vi "Get IO Nodes.vi"(8 "error in (no error)":errorcluster, 11 "DAQ in":refnum<class "DAQ.lvclass">) -> (0 "error out":errorcluster, 2 "IO Nodes":T1 {"AO Config"."AO Channels"."Conversion"."ScaleOffset" format="%.3f"; "AO Config"."AO Channels"."Conversion"."MinEngUnit" format="%.3f"; "AO Config"."AO Channels"."Conversion"."MaxEngUnit" format="%.3f"; "AO Config"."AO Channels"."Conversion"."MinSignal" format="%.3f"; "AO Config"."AO Channels"."Conversion"."MaxSignal" format="%.3f"; "AI Config"."AI Tasks"."AI Channels"."Conversion"."ScaleOffset" format="%.3f"; "AI Config"."AI Tasks"."AI Channels"."Conversion"."MinEngUnit" format="%.3f"; "AI Config"."AI Tasks"."AI Channels"."Conversion"."MaxEngUnit" format="%.3f"; "AI Config"."AI Tasks"."AI Channels"."Conversion"."MinSignal" format="%.3f"; "AI Config"."AI Tasks"."AI Channels"."Conversion"."MaxSignal" format="%.3f"; "AI Config"."AI Tasks"."AI Channels"."Terminal Configuration" items=["default"=-1, "RSE"=10083, "NRSE"=10078, "Differential"=10106, "Pseudodifferential"=12529]}, 3 "DAQ out":refnum<class "DAQ.lvclass">)   [LabVIEW 2017, in "DAQ.lvclass"]
doc: "Developed by Kevin Thompson\nkevin@thompsonengineering.net\n\nCopyright 2018-2020\nThompson Engineering, LLC"
uses:
  DAQ.lvclass
  DataTypes/TD IO Node Definition--cluster.ctl
  DataTypes/TD DI Config--cluster.ctl
  DataTypes/TD DI Task--cluster.ctl
  DataTypes/TD DI Channel--cluster.ctl
  DataTypes/TD DO Config--cluster.ctl
  DataTypes/TD DO Channel--cluster.ctl
  DataTypes/TD AI Config--cluster.ctl
  DataTypes/TD AI Task--cluster.ctl
  DataTypes/TD AI Channel--cluster.ctl
  DataTypes/TD DataValueConversion--cluster.ctl
  DataTypes/TD AI DAQ Type--enum.ctl
  DataTypes/TD AI Force Bridge--cluster.ctl
  DataTypes/TD AO Config--cluster.ctl
  DataTypes/TD AO Channel--cluster.ctl
  DAQ.lvclass/DAQ.ctl
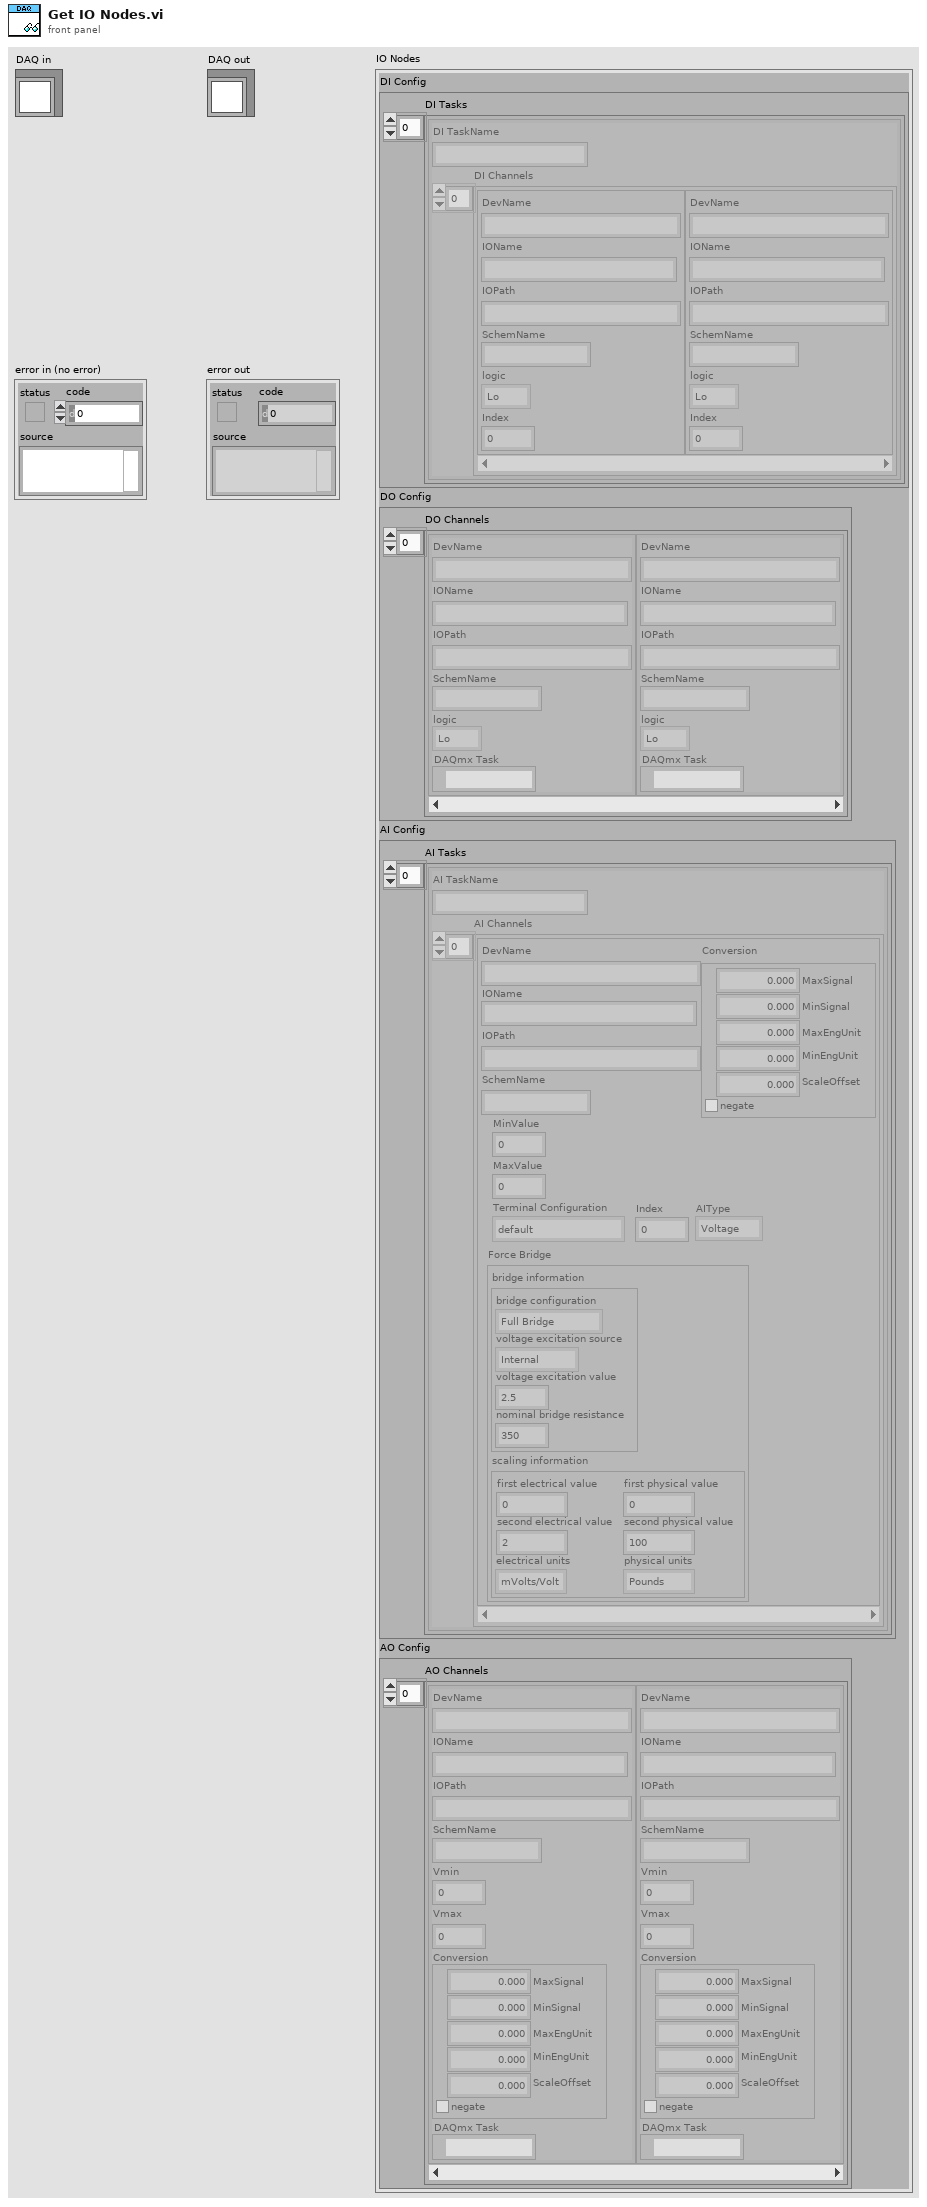
[diagram p1: front panel]
types:
  T1 = typedef "DAQ.lvclass/TD IO Node Definition--cluster.ctl" = cluster{"DI Config":T2, "DO Config":T5, "AI Config":T7, "AO Config":T13}
  T2 = typedef "DAQ.lvclass/TD DI Config--cluster.ctl" = cluster{"DI Tasks":T3[]}
  T3 = typedef "DAQ.lvclass/TD DI Task--cluster.ctl" = cluster{"DI TaskName":string, "DI Channels":T4[]}
  T4 = typedef "DAQ.lvclass/TD DI Channel--cluster.ctl" = cluster{"DevName":string, "IOName":string, "IOPath":string, "SchemName":string, "logic":enum16{"Lo", "Hi"}, "Index":i32}
  T5 = typedef "DAQ.lvclass/TD DO Config--cluster.ctl" = cluster{"DO Channels":T6[]}
  T6 = typedef "DAQ.lvclass/TD DO Channel--cluster.ctl" = cluster{"DevName":string, "IOName":string, "IOPath":string, "SchemName":string, "logic":enum16{"Lo", "Hi"}, "DAQmx Task":refnum<k21>}
  T7 = typedef "DAQ.lvclass/TD AI Config--cluster.ctl" = cluster{"AI Tasks":T8[]}
  T8 = typedef "DAQ.lvclass/TD AI Task--cluster.ctl" = cluster{"AI TaskName":string, "AI Channels":T9[]}
  T9 = typedef "DAQ.lvclass/TD AI Channel--cluster.ctl" = cluster{"DevName":string, "IOName":string, "IOPath":string, "SchemName":string, "MinValue":dbl, "MaxValue":dbl, "Terminal Configuration":i32, "Index":i32, "Conversion":T10, "AIType":T11, "Force Bridge":T12}
  T10 = typedef "DAQ.lvclass/TD DataValueConversion--cluster.ctl" = cluster{"MaxSignal":dbl, "MinSignal":dbl, "MaxEngUnit":dbl, "MinEngUnit":dbl, "ScaleOffset":dbl, "negate":bool}
  T11 = typedef "DAQ.lvclass/TD AI DAQ Type--enum.ctl" = enum16{"Voltage", "Current", "Strain Gage", "Force Bridge"}
  T12 = typedef "DAQ.lvclass/TD AI Force Bridge--cluster.ctl" = cluster{"bridge information":cluster{"bridge configuration":i32, "voltage excitation source":i32, "voltage excitation value":dbl, "nominal bridge resistance":dbl}, "scaling information":cluster{"first electrical value":dbl, "second electrical value":dbl, "electrical units":i32, "first physical value":dbl, "second physical value":dbl, "physical units":i32}}
  T13 = typedef "DAQ.lvclass/TD AO Config--cluster.ctl" = cluster{"AO Channels":T14[]}
  T14 = typedef "DAQ.lvclass/TD AO Channel--cluster.ctl" = cluster{"DevName":string, "IOName":string, "IOPath":string, "SchemName":string, "Vmin":dbl, "Vmax":dbl, "Conversion":T10, "DAQmx Task":refnum<k21>}
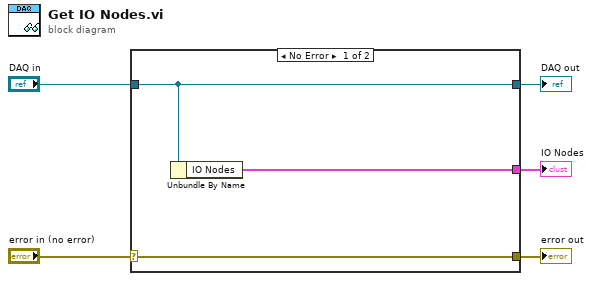
[diagram p0: block diagram]
diagram:
  n1 = case shown="No Error" "error in (no error)" {
    selector: "error in (no error)" -> [w8 w9]
    tunnel: [w8 w9] -> w4
    tunnel: [w7 w10] -> w2
    tunnel: "DAQ in" -> [w7 w10]
    tunnel: [w6 _] -> w1
    frame No Error {
      n2 = Unbundle By Name(w7) -> ("IO Nodes"=w6:T1)
    }
    frame Error {
    }
  }
  "error out" <- w4
  "DAQ out" <- w2
  "IO Nodes" <- w1
